vi "GetTimestampFormat.vi"(8 "Error in (no error)":errorcluster, 11 "Log in":refnum<class "Log.lvclass">) -> (0 "Error out":errorcluster, 2 "TimestampFormat":string, 3 "Log out":refnum<class "Log.lvclass">)   [LabVIEW 2011, in "Log.lvclass"]
uses:
  Log.lvclass
  Log.lvclass/Log.ctl
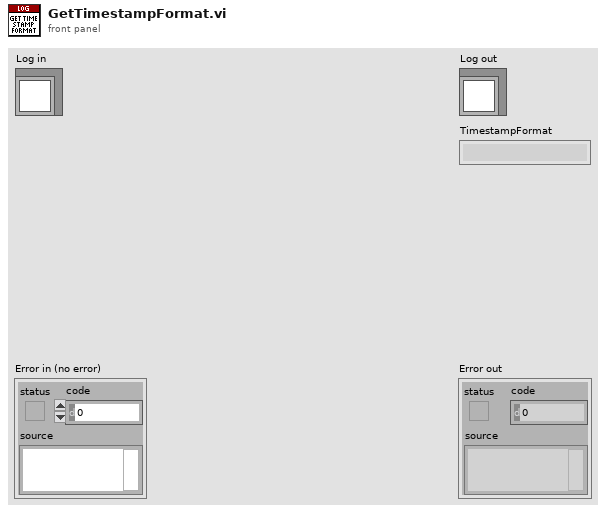
[diagram p1: front panel]
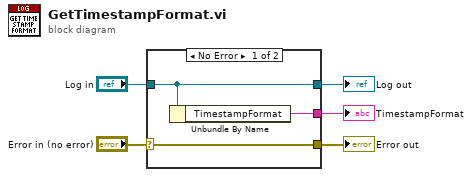
[diagram p0: block diagram]
diagram:
  n1 = case shown="No Error" "Error in (no error)" {
    selector: "Error in (no error)" -> [w8 w9]
    tunnel: [w8 w9] -> w4
    tunnel: [w7 w10] -> w2
    tunnel: "Log in" -> [w7 w10]
    tunnel: [w6 _] -> w1
    frame No Error {
      n2 = Unbundle By Name(w7) -> ("TimestampFormat"=w6:string)
    }
    frame Error {
    }
  }
  "Error out" <- w4
  "Log out" <- w2
  "TimestampFormat" <- w1
